vi "ConvertStringToTriggerSource.vi"(11 "Trigger Source String":string) -> (3 "Trigger Source":T1)   [LabVIEW 2012, in "Keithley-7001.lvlib"]
uses:
  Keithley-7001.lvlib
  Public/Controls/TriggerSource.ctl
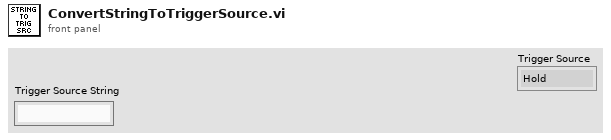
[diagram p1: front panel]
types:
  T1 = typedef "Keithley-7001.lvlib/TriggerSource.ctl" = enum16{"Hold", "Immediate", "Manual", "Bus", "External", "Timer"}
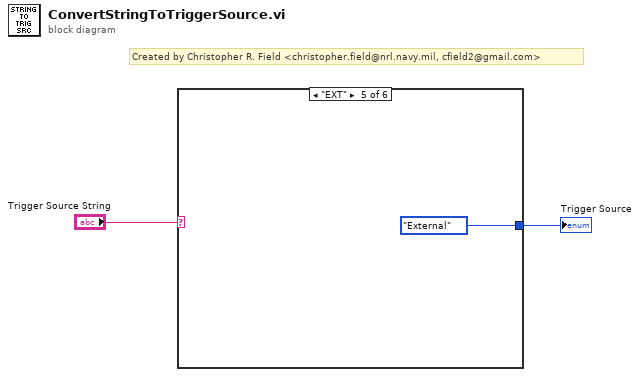
[diagram p0: block diagram]
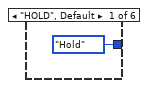
[diagram p2: hidden frame]
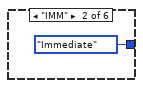
[diagram p3: hidden frame]
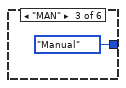
[diagram p4: hidden frame]
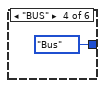
[diagram p5: hidden frame]
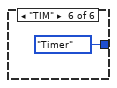
[diagram p6: hidden frame]
diagram:
  # "Created by Christopher R. Field <christopher.field@nrl.navy.mil, cfield2@gmail.com>"
  n1 = case shown="\"EXT\"" "Trigger Source String" {
    tunnel: [TriggerSource."Hold" ("Trigger Source") TriggerSource."Immediate" ("Trigger Source") TriggerSource."Manual" ("Trigger Source") TriggerSource."Bus" ("Trigger Source") TriggerSource."External" ("Trigger Source") TriggerSource."Timer" ("Trigger Source")] -> w1
    frame "HOLD", Default {
    }
    frame "IMM" {
    }
    frame "MAN" {
    }
    frame "BUS" {
    }
    frame "EXT" {
    }
    frame "TIM" {
    }
  }
  "Trigger Source" <- w1
